vi "SDCP SMF Rx Logger - Base.vi"() -> ()   [LabVIEW 2020]
uses:
  Typedefs/SDCP SMF logger - SMF with timestamp.ctl
  Typedefs/SDCP SMF Rx Logger - Notifier FGV - Notifier names.ctl
  Typedefs/SDCP SMF Rx Logger - Notifier FGV - Commands.ctl
  Typedefs/SDCP - Serial Port Control - Commands.ctl
panel:
  out "Logged data":T1[](array[typedef])
  out "error out":errorcluster
  in  "error in (no error)":errorcluster
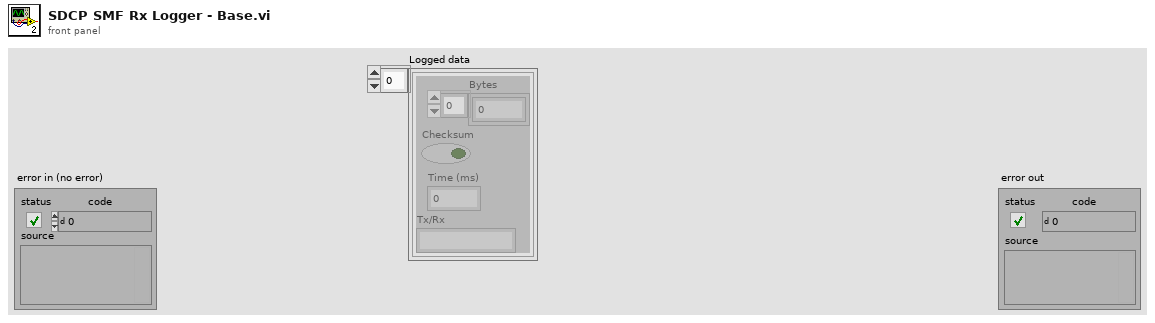
[diagram p1: front panel]
types:
  T1 = typedef "SDCP SMF logger - SMF with timestamp.ctl" = cluster{"Bytes":u8[], "Checksum":bool, "Time (ms)":u32, "Tx/Rx":string}
  T2 = typedef "SDCP SMF Rx Logger - Notifier FGV - Commands.ctl" = enum16{"Initialize", "Read", "Write", "Deinitialize"}
  T3 = typedef "SDCP SMF Rx Logger - Notifier FGV - Notifier names.ctl" = enum16{"Logged data", "Pause logging", "Get log", "Reset log", "Sample counter", "Logged data buffer", "Stop logging"}
  T4 = typedef "SDCP - Serial Port Control - Commands.ctl" = enum16{"Open", "Read", "Write", "Get instance", "Close"}
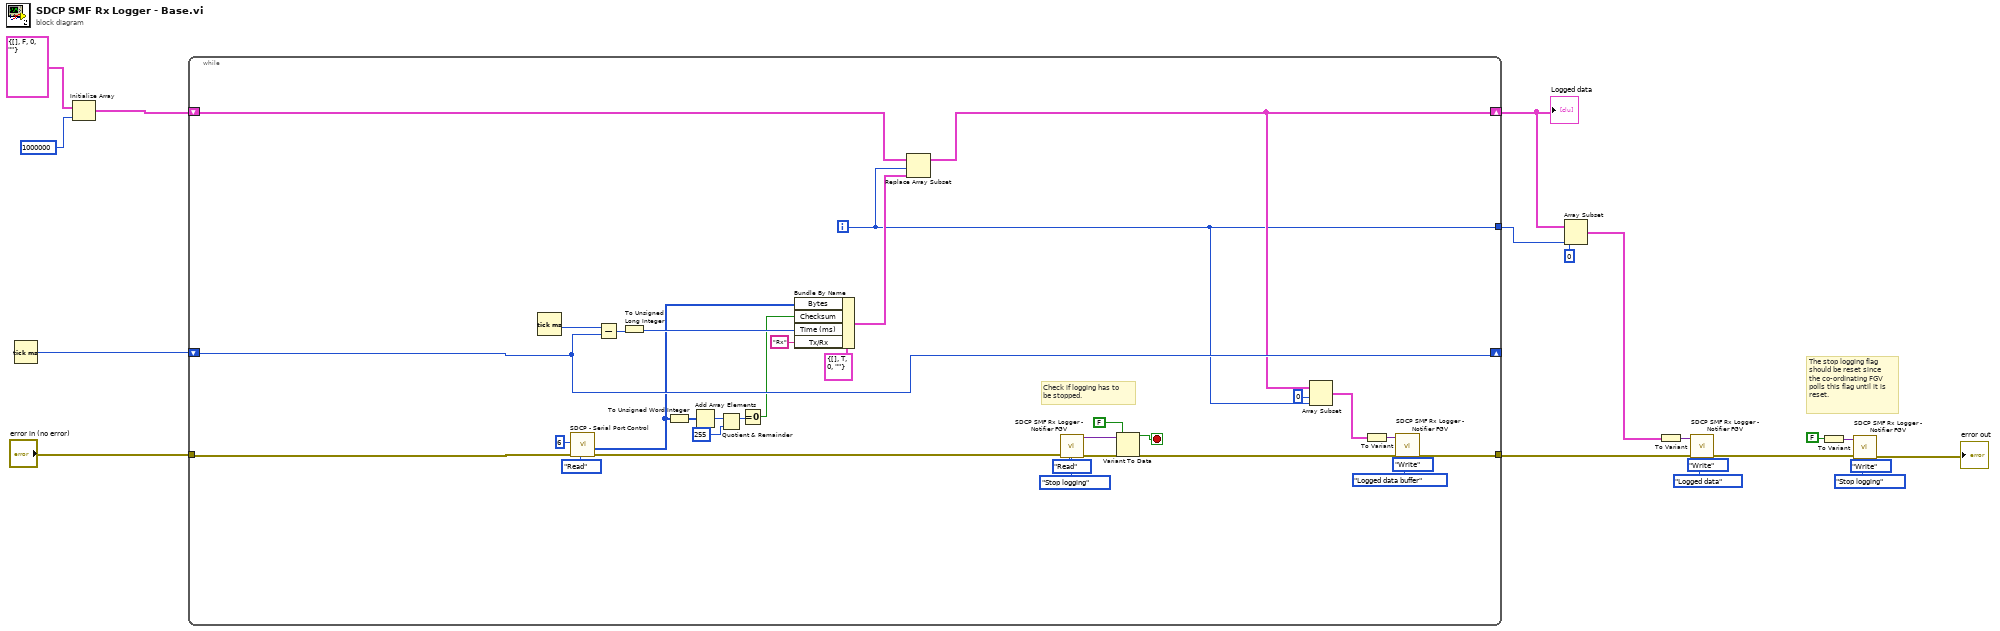
[diagram p0: block diagram]
diagram:
  # "The stop logging flag\nshould be reset since\nthe co-ordinating FGV\npolls this flag until it is\nreset."
  n1 = Tick Count (ms)() -> (millisecond timer value=w19:u32)
  n2 = Initialize Array(T1 {"Bytes"=[], "Checksum"=FALSE, "Time (ms)"=0, "Tx/Rx"=""} ("SMF with timestamp"), 1000000 ("dimension size")) -> (w12:T1[])
  n3 = while {
    tunnel: "error in (no error)" -> [w29]
    shift-right: [w52] -> _
    shift-left: w19 -> [w52]
    tunnel: [w24] -> w6
    shift-right: [w23] -> w4
    shift-left: w12 -> [w44]
    tunnel: [w21] -> w2
    i -> [w21]
    stop <- w45 stop-if-true
    # "Check if logging has to\nbe stopped."
    n4 = Tick Count (ms)() -> (millisecond timer value=w40:u32)
    n5 = call "SDCP - Serial Port Control.vi"("Command"=SDCP_-_Serial_Port_Control_-_Commands."Read", "error in (no error)"=w29, "Read byte count"=u32 6) -> ("error out"=w46:errorcluster, "Received bytes"=w36:u8[])  [unwired: 7 in]
    n6 = Subtract(x=w40, y=w52) -> (x-y=w39:u32)
    n7 = To Unsigned Long Integer(number=w39) -> (unsigned 32bit integer=w38:u32)
    n8 = To Unsigned Word Integer(number=w36) -> (unsigned 16bit integer=w35:u16[])
    n9 = Add Array Elements(numeric array=w35) -> (sum=w34:u16)
    n10 = Quotient & Remainder(x=w34, y=u16 255) -> (x-y*floor(x/y)=w32:u16)  [unwired: 1 out]
    n11 = Equal To 0?(x=w32) -> (x = 0?=w31:bool)
    n12 = Bundle By Name(cluster=T1 {"Bytes"=[], "Checksum"=TRUE, "Time (ms)"=0, "Tx/Rx"=""} ("SMF with timestamp"), "Bytes"=w36, "Checksum"=w31, "Time (ms)"=w38, "Tx/Rx"="Rx") -> (w30:T1)
    n13 = Replace Array Subset(array=w44, new element=w30, index=w21) -> (w23:T1[])
    n14 = call "SDCP SMF Rx Logger - Notifier FGV.vi"("error in (no error)"=w46, "Command"=SDCP_SMF_Rx_Logger_-_Notifier_FGV_-_Commands."Read", "Notifier name"=SDCP_SMF_Rx_Logger_-_Notifier_FGV_-_Notifier_names."Stop logging") -> ("error out"=w51:errorcluster, "Notifier value out"=w50:variant)  [unwired: 3 in]
    n15 = Variant To Data(error in=w51, type=FALSE, Variant=w50) -> (data=w45:bool, error out=w25:errorcluster)
    n16 = Array Subset(array=w23, index=0, length=w21) -> (w22:T1[])
    n17 = To Variant(anything=w22) -> (Variant=w28:variant)
    n18 = call "SDCP SMF Rx Logger - Notifier FGV.vi"("error in (no error)"=w25, "Command"=SDCP_SMF_Rx_Logger_-_Notifier_FGV_-_Commands."Write", "Notifier name"=SDCP_SMF_Rx_Logger_-_Notifier_FGV_-_Notifier_names."Logged data buffer", "Notifier value in"=w28) -> ("error out"=w24:errorcluster)  [unwired: 2 in, 1 out]
  }
  "Logged data" <- w4
  n19 = Array Subset(array=w4, index=0, length=w2) -> (w1:T1[])
  n20 = To Variant(anything=w1) -> (Variant=w9:variant)
  n21 = call "SDCP SMF Rx Logger - Notifier FGV.vi"("error in (no error)"=w6, "Command"=SDCP_SMF_Rx_Logger_-_Notifier_FGV_-_Commands."Write", "Notifier name"=SDCP_SMF_Rx_Logger_-_Notifier_FGV_-_Notifier_names."Logged data", "Notifier value in"=w9) -> ("error out"=w5:errorcluster)  [unwired: 2 in, 1 out]
  n22 = To Variant(anything=FALSE) -> (Variant=w18:variant)
  n23 = call "SDCP SMF Rx Logger - Notifier FGV.vi"("error in (no error)"=w5, "Command"=SDCP_SMF_Rx_Logger_-_Notifier_FGV_-_Commands."Write", "Notifier name"=SDCP_SMF_Rx_Logger_-_Notifier_FGV_-_Notifier_names."Stop logging", "Notifier value in"=w18) -> ("error out"=→"error out":errorcluster)  [unwired: 2 in, 1 out]
